vi "WPI_ERRSetOnNotAllocatedRelay.vi"(8 "error in (no error)":errorcluster, 10 "Relay Channel":T1) -> (0 "error out":errorcluster)   [LabVIEW 2017]
doc: "This software is licensed. Open the labview\\readme\\WPI Robotics Library Open Source License.txt file for more information."
uses:
  <vilib>/Rock Robotics/SystemInterfaces/DIO/FPGA_DIORelayChannel.ctl
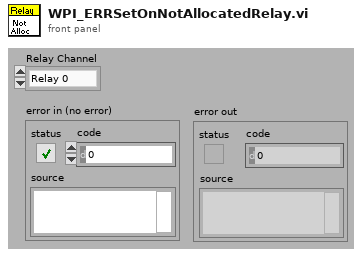
[diagram p1: front panel]
types:
  T1 = typedef "FPGA_DIORelayChannel.ctl" = enum8{"Relay 0", "Relay 1", "Relay 2", "Relay 3", "Invalid"}
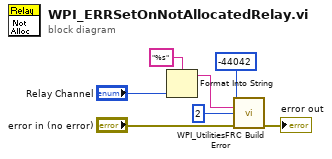
[diagram p0: block diagram]
diagram:
  n1 = Format Into String(format string="%s", "Relay Channel") -> (resulting string=w6:string)  [unwired: 2 in, 1 out]
  n2 = call <vilib>:"WPI_UtilitiesFRC Build Error.vi"("error code"=-44042 ("code"), "extra error text"=w6, "chain levels to remove (1)"=2, "error in (no error)"="error in (no error)") -> ("error out"=→"error out":errorcluster)  [unwired: 1 in, 10 out]
